vi "Controller Process.vi"(8 "error in (no error)":errorcluster, 11 "View Model":T1) -> (0 "error out":errorcluster)   [LabVIEW 2017]
doc: "Controller process is a central part of application. Operate all requests from all other processes."
uses:
  View Model/Controls/View Model.ctl
  View Model/Controls/Shared Model.ctl
  Error Handler/Controls/Error Model.ctl
  Error Handler/Controls/Error Event.ctl
  Error Handler/Controls/Error Type.ctl
  Controls/Controller Model.ctl
  Controls/Controller Event.ctl
  Controls/Controller Command.ctl
  Controls/Controller Overhead.ctl
  Real-Time/RT Status.ctl
  Real-Time/RT Loop Status.ctl
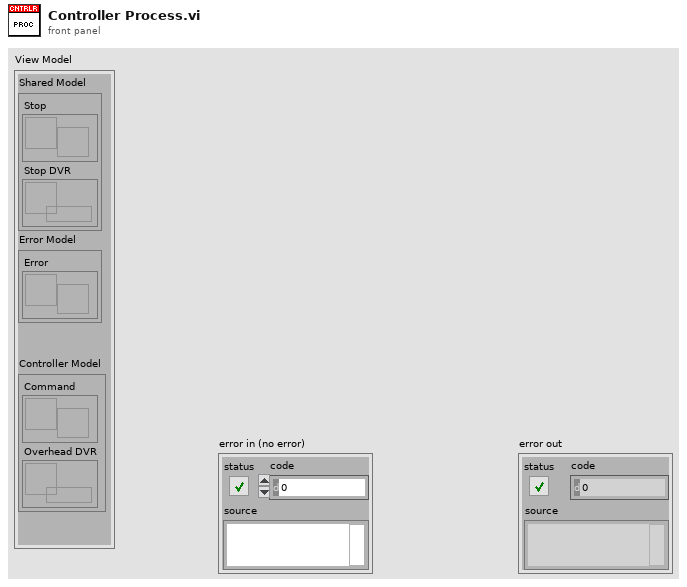
[diagram p1: front panel]
types:
  T1 = typedef "View Model.ctl" = cluster{"Shared Model":T2, "Error Model":T3, "Controller Model":T4}
  T2 = typedef "Shared Model.ctl" = cluster{"Stop":refnum<user-event>, "Stop DVR":refnum<data-value>}
  T3 = typedef "Error Model.ctl" = cluster{"Error":refnum<user-event>}
  T4 = typedef "Controller Model.ctl" = cluster{"Command":refnum<user-event>, "Overhead DVR":refnum<data-value>}
  T5 = typedef "Error Type.ctl" = enum16{"Minor", "Critical"}
  T6 = typedef "RT Status.ctl" = cluster{"Status TCL1":T7, "Status TCL2":T7, "Status NPL":T7, "Connected?":bool}
  T7 = typedef "RT Loop Status.ctl" = cluster{"Duration, us":dbl, "Late Counter":i32, "Timeout, us":u32}
  T8 = typedef "Controller Command.ctl" = enum16{"Idle", "Init", "Stop App", "Stop RT"}
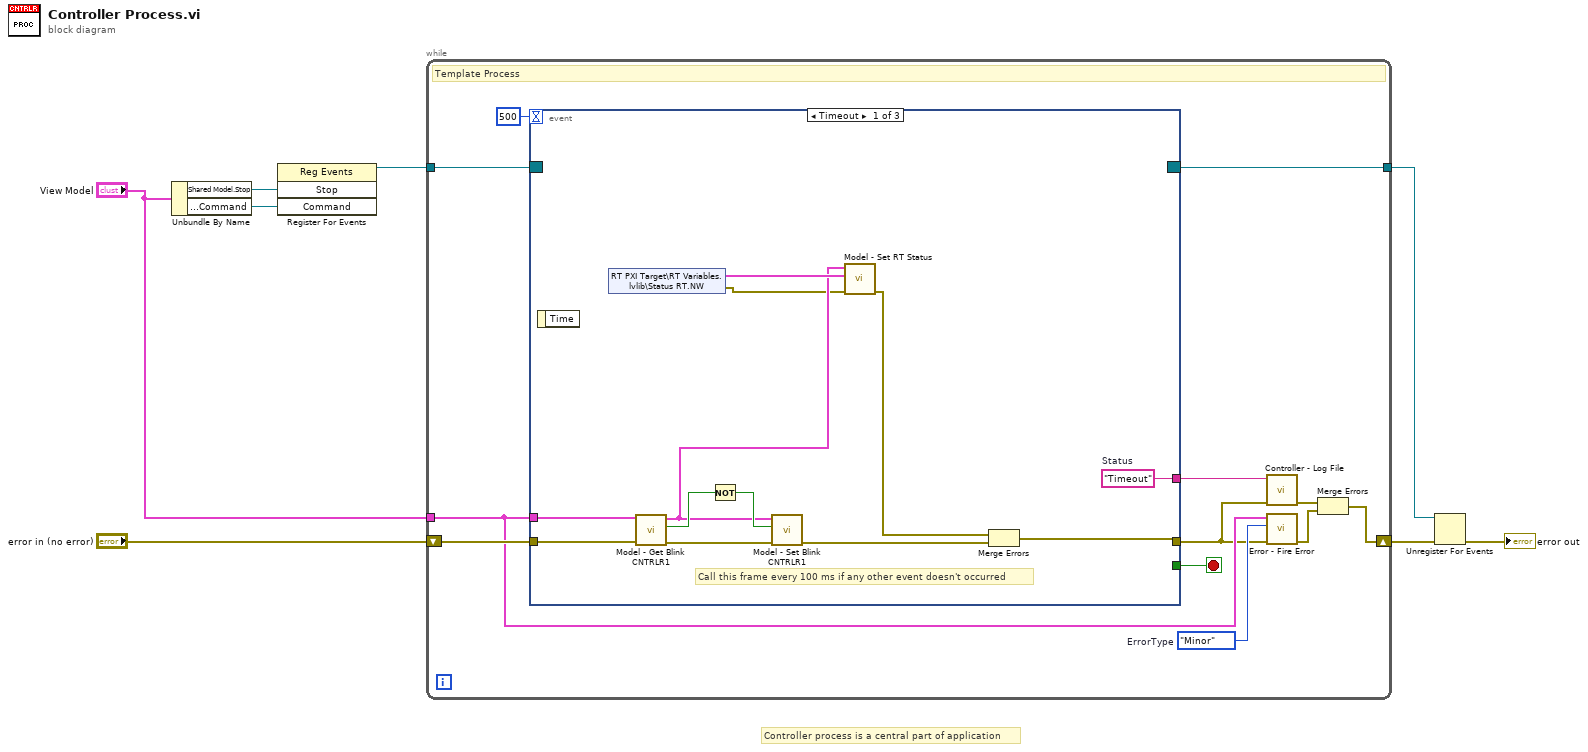
[diagram p0: block diagram]
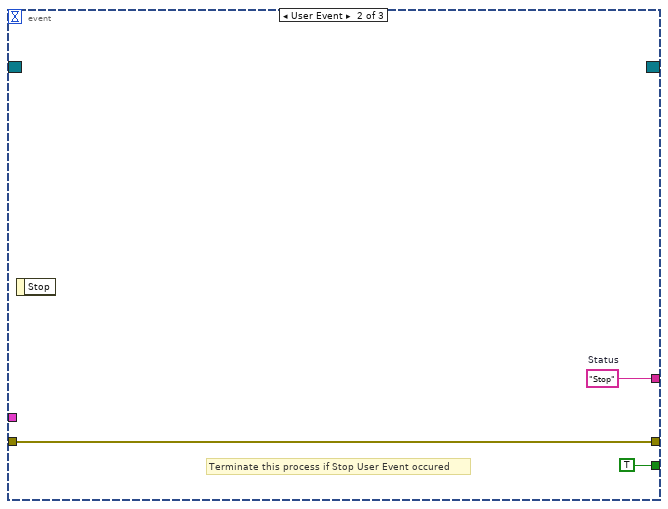
[diagram p2: hidden frame]
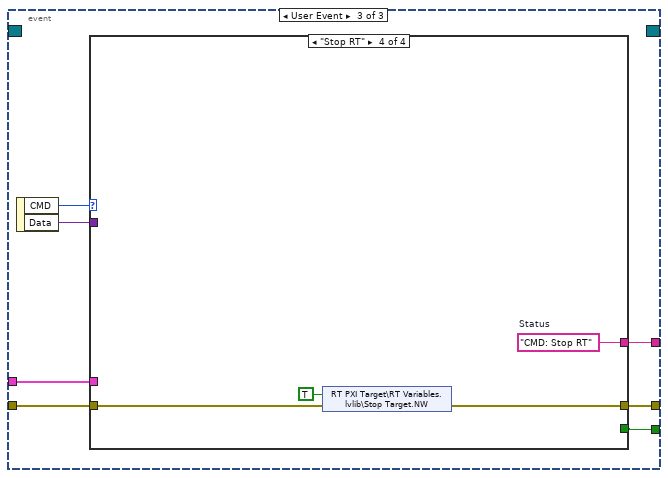
[diagram p3: hidden frame]
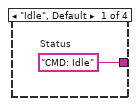
[diagram p4: hidden frame]
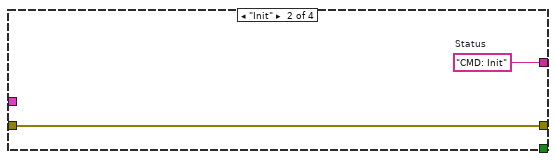
[diagram p5: hidden frame]
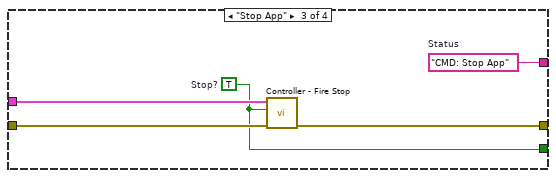
[diagram p6: hidden frame]
diagram:
  # "Controller process is a central part of application"
  n1 = Unbundle By Name("View Model") -> ("Shared Model.Stop"=w8:refnum<user-event>, "Controller Model.Command"=w1:refnum<user-event>)
  n2 = register-events(w8, w1) -> (reference out=w7:refnum<event-registration>)  [unwired: 2 in, 1 out]
  n3 = while {
    tunnel: w7 -> [w18]
    shift-right: [w10] -> w4
    shift-left: "error in (no error)" -> [w20]
    tunnel: "View Model" -> [w15]
    tunnel: [w17] -> w3
    stop <- w16 stop-if-true
    w14 = Error_Type."Minor"  # ErrorType
    # "Template Process"
    n4 = event shown="[0] Timeout" {
      selector: w18 -> [_ _ _]
      dyn-events: [_ _ _] -> w17
      timeout: 500 -> [_ _ _]
      tunnel: w20 -> [w25 w35 w39]
      tunnel: w15 -> [w32 _ w40]
      tunnel: [w27 w35 w38] -> w13
      tunnel: [_ TRUE w37] -> w16
      tunnel: [w26 w33 w36] -> w9
      event Timeout {
        w26 = "Timeout"  # Status
        # "Call this frame every 100 ms if any other event doesn't occurred"
        n5 = event-data() -> ()  [unwired: 1 in, 1 out]
        n6 = shared-variable "RT PXI Target\\RT Variables.lvlib\\Status RT.NW"() -> (w24:T6, error out=w22:errorcluster)  [unwired: 1 in]
        n7 = call "Model - Get Blink CNTRLR1.vi"("error in (no error)"=w25, "View Model"=w32) -> ("error out"=w29:errorcluster, "BlinkC1"=w31:bool, "View Model"=w23:T1)  [unwired: 7 in]
        n8 = Not(x=w31) -> (.not. x?=w30:bool)
        n9 = call "Model - Set Blink CNTRLR1.vi"("error in (no error)"=w29, "BlinkC1"=w30, "View Model"=w23) -> ("error out"=w28:errorcluster)  [unwired: 7 in, 1 out]
        n10 = call "Model - Set RT Status.vi"("error in (no error)"=w22, "RT Status"=w24, "View Model"=w23) -> ("error out"=w21:errorcluster)  [unwired: 7 in, 1 out]
        n11 = Merge Errors(w21, w28) -> (w27:errorcluster)
      }
      event User Event {
        w33 = "Stop"  # Status
        # "Terminate this process if Stop User Event occured"
        n12 = event-data() -> ()  [unwired: 1 in, 1 out]
      }
      event User Event {
        n13 = event-data() -> ("CMD"=w42:T8, "Data"=w41:variant)  [unwired: 1 in]
        n14 = case shown="\"Stop RT\"" w42 {
          tunnel: w41 -> [_ _ _ _]
          tunnel: w40 -> [_ _ w49 _]
          tunnel: w39 -> [_ w45 w50 w53]
          tunnel: [_ w45 w48 w52] -> w38
          tunnel: [_ _ w47 _] -> w37
          tunnel: [w43 w44 w46 w54] -> w36
          frame "Idle", Default {
            w43 = "CMD: Idle"  # Status
          }
          frame "Init" {
            w44 = "CMD: Init"  # Status
          }
          frame "Stop App" {
            w46 = "CMD: Stop App"  # Status
            w47 = TRUE  # Stop?
            n15 = call "Controller - Fire Stop.vi"("error in (no error)"=w50, "Stop?"=w47, "View Model"=w49) -> ("error out"=w48:errorcluster)  [unwired: 8 in]
          }
          frame "Stop RT" {
            w54 = "CMD: Stop RT"  # Status
            n16 = shared-variable "RT PXI Target\\RT Variables.lvlib\\Stop Target.NW"(TRUE ("Stop Target.NW"), error in=w53) -> (error out=w52:errorcluster)
          }
        }
      }
    }
    n17 = call "Controller - Log File.vi"("error in"=w13, "Status"=w9) -> ("error out"=w12:errorcluster)  [unwired: 9 in]
    n18 = call "Error - Fire Error.vi"("error in (no error)"=w13, "ErrorType"=w14, "View Model"=w15) -> ("error out"=w11:errorcluster)  [unwired: 7 in, 1 out]
    n19 = Merge Errors(w12, w11) -> (w10:errorcluster)
  }
  n20 = Unregister For Events(event registration refnum=w3, error in=w4) -> (error out=→"error out":errorcluster)
